vi "Amira Bladder Calibration V0.2.vi"() -> ()   [LabVIEW 2020]
uses:
  <userlib>/KQD LabVIEW User/Serial/Controls/SERIAL PortConfig.ctl
  <userlib>/KQD LabVIEW User/Serial/Controls/SERIAL BaudRate.ctl
  <userlib>/Amira UART/Amira UART.lvclass
  <userlib>/KQD LabVIEW User/Serial/Serial.lvlib
panel:
  out "Data":dbl[][](graph)
  in  "Iteration":i32=1
  in  "RunWith":cluster{"Steps":i32, "Rates":i32}={"Steps"=400, "Rates"=40}
  in  "Folder":path=path "C:/Amira Data/Strip"
  in  "StartAt":cluster{"Steps":i32, "Rates":i32}={"Steps"=950, "Rates"=200}
  out "Position":dbl[](graph)
  in  "DAQ":tag="Dev1/port0"
  out "UART":string
  in  "ComPort":refnum<visa-resource-name>
  in  "Config":T1={"BaudRate"=enum."460800", "StopBits"=10, "DataBits"=8, "Parity"=enum."None", "FlowControl"=2, "TimeOut"=1000, "TermChar"=10, "ReadTermEn"=TRUE} {"TermChar" format="%.0x"; "FlowControl" items=["None", "XON/XOFF", "RTS/CTS", "XON/XOFF & RTS/CTS", "DTR/DSR", "XON/XOFF & DTR/DSR"]; "DataBits" min=5 max=8 step=1; "StopBits" items=["1.0"=10, "1.5"=15, "2.0"=20]}
  out "ErrOut":errorcluster
  in  "ErrIn":errorcluster
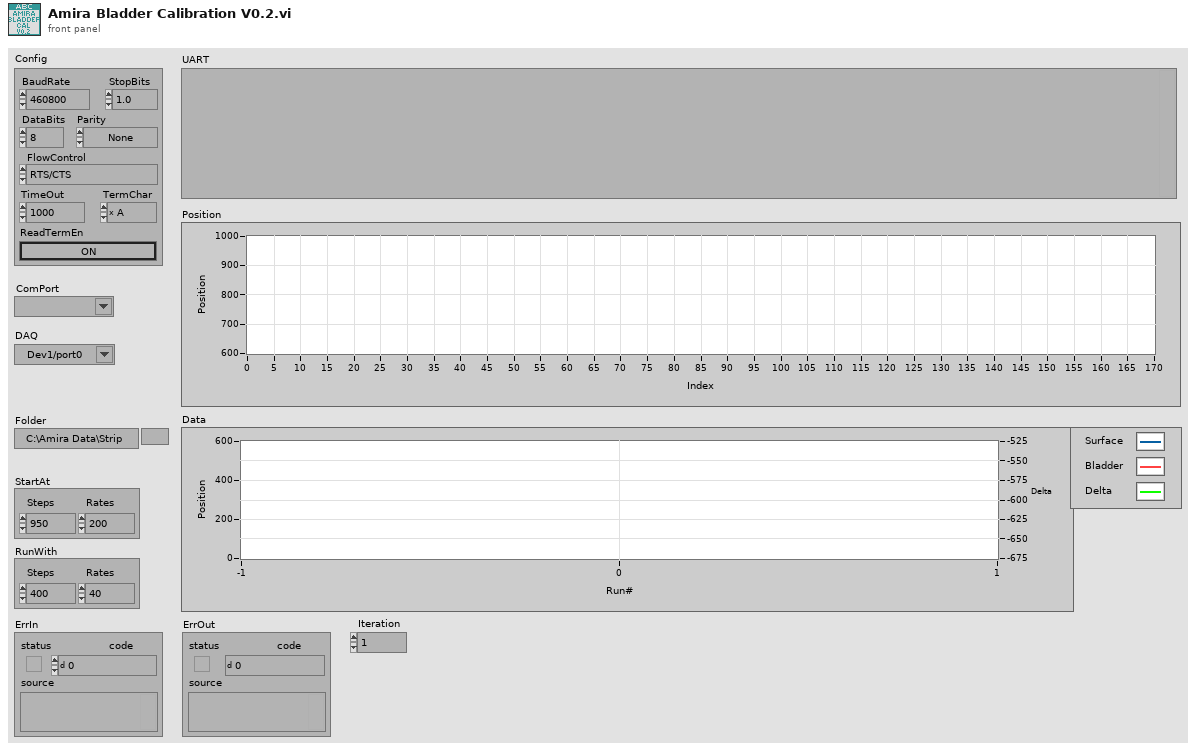
[diagram p1: front panel]
types:
  T1 = typedef "Serial.lvlib/SERIAL PortConfig.ctl" = cluster{"BaudRate":T2, "StopBits":u16, "DataBits":u16, "Parity":enum16{"None", "Odd", "Even", "Mark", "Space"}, "FlowControl":u16, "TimeOut":u32, "TermChar":u8, "ReadTermEn":bool}
  T2 = typedef "SERIAL BaudRate.ctl" = enum16{"2400", "4800", "7200", "9600", "14400", "19200", "28800", "38400", "57600", "115200", "128000", "230400", "460800", "921600"}
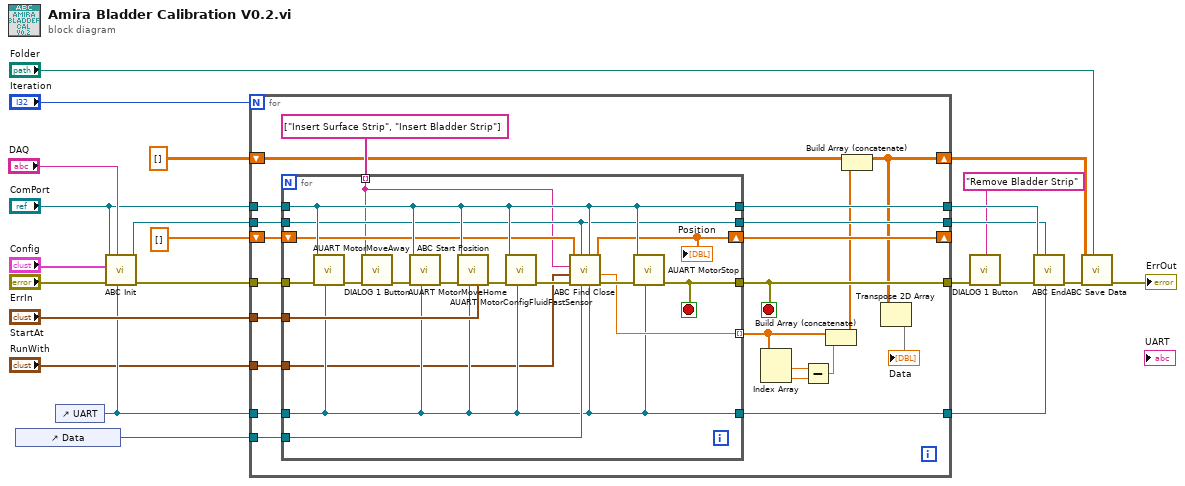
[diagram p0: block diagram]
diagram:
  n1 = control-ref of="Data"() -> (w18:refnum<vi>)
  n2 = control-ref of="UART"() -> (w16:refnum<vi>)
  n3 = call "ABC Init.vi"("UART"=w16, "DAQ"="DAQ", "ErrIn"="ErrIn", "PortConfig"="Config", "ComPort"="ComPort") -> ("ErrOut"=w17:errorcluster, "DaqTask"=w19:refnum<k21>)  [unwired: 5 in]
  n4 = for {
    N: "Iteration" -> [_]
    tunnel: "StartAt" -> [w45]
    tunnel: w18 -> [w43]
    tunnel: "ComPort" -> [w40]
    tunnel: [w38] -> w14
    tunnel: w19 -> [w44]
    tunnel: [w37] -> w13
    tunnel: w17 -> [w42]
    tunnel: [w33] -> w3
    tunnel: w16 -> [w41]
    tunnel: [w35] -> w11
    shift-right: [w34] -> _
    shift-left: dbl[] [] ("DataOut") -> [w36]
    shift-right: [w27] -> w6
    shift-left: dbl[][] [] -> [w26]
    tunnel: "RunWith" -> [w24]
    stop <- w33 stop-if-true
    n5 = for {
      tunnel: w45 -> [w61]
      tunnel: w44 -> [w56]
      tunnel: w43 -> [w59]
      tunnel: w41 -> [w52]
      tunnel: w40 -> [w57]
      tunnel: w42 -> [w48]
      tunnel: [w58] -> w33
      tunnel: string[] ["Insert Surface Strip", "Insert Bladder Strip"] -> [w49] mode=indexing
      tunnel: [w57] -> w38
      tunnel: [w56] -> w37
      shift-right: [w55] -> w34
      shift-left: w36 -> [w54]
      tunnel: [w53] -> w32 mode=indexing
      tunnel: [w52] -> w35
      tunnel: w24 -> [w50]
      stop <- w58 stop-if-true
      n6 = call <userlib>:"AUART MotorMoveAway.vi"("UART"=w52, "ErrIn"=w48, "Port"=w57) -> ("ErrOut"=w47:errorcluster)  [unwired: 8 in]
      n7 = call <userlib>:"DIALOG 1 Button.vi"("ErrIn"=w47, "Msg"=w49) -> ("ErrOut"=w46:errorcluster)  [unwired: 9 in]
      n8 = call <userlib>:"AUART MotorMoveHome.vi"("UART"=w52, "ErrIn"=w46, "Port"=w57) -> ("ErrOut"=w63:errorcluster)  [unwired: 7 in, 1 out]
      n9 = call "ABC Start Position.vi"("Start"=w61, "UART"=w52, "ErrIn"=w63, "ComPort"=w57) -> ("ErrOut"=w62:errorcluster)  [unwired: 6 in, 1 out]
      n10 = call <userlib>:"AUART MotorConfigFluidFastSensor.vi"("UART"=w52, "ErrIn"=w62, "Port"=w57) -> ("ErrOut"=w51:errorcluster)  [unwired: 8 in]
      n11 = call "ABC Find Close.vi"("UART"=w52, "ComPort"=w57, "Data"=w59, "DaqTask"=w56, "ErrIn"=w51, "RunWith"=w50, "Strip"=w49, "DataIn"=w54) -> ("ErrOut"=w60:errorcluster, "FrontClose"=w53:dbl, "DataOut"=w55:dbl[])  [unwired: 1 in]
      "Position" <- w55
      n12 = call <userlib>:"AUART MotorStop.vi"("UART"=w52, "ErrIn"=w60, "Port"=w57) -> ("ErrOut"=w58:errorcluster)  [unwired: 7 in, 1 out]
    }
    n13 = Index Array(array=w32) -> (element #1=w31:dbl, element #2=w30:dbl)  [unwired: 2 in]
    n14 = Subtract(x=w31, y=w30) -> (x-y=w29:dbl)
    n15 = Build Array (concatenate)(w32, w29) -> (w28:dbl[])
    n16 = Build Array (concatenate)(w26, w28) -> (w27:dbl[][])
    n17 = Transpose 2D Array(2D array=w27) -> (transposed array=→"Data":dbl[][])
  }
  n18 = call <userlib>:"DIALOG 1 Button.vi"("ErrIn"=w3, "Msg"="Remove Bladder Strip") -> ("ErrOut"=w2:errorcluster)  [unwired: 9 in]
  n19 = call "ABC End.vi"("UART"=w11, "DaqTask"=w13, "ErrIn"=w2, "ComPort"=w14) -> ("ErrOut"=w7:errorcluster)  [unwired: 7 in]
  n20 = call "ABC Save Data.vi"("Folder"="Folder", "ErrIn"=w7, "Data"=w6) -> ("ErrOut"=→"ErrOut":errorcluster)  [unwired: 8 in]
